vi "Actor Receive.vi"(11 "Process in":refnum<class "ABD.lvclass">) -> (0 "error out":errorcluster, 2 "Msg":refnum<class "Msg Strategy.lvclass">)   [LabVIEW 2021, in "ABD.lvlib" / "ABD.lvclass"]
uses:
  ABD.lvclass
  LVCAM/LVCAM/Msg Strategy/Msg Strategy.lvclass
  ABD.lvclass/ABD.ctl
  LVCAM/LVCAM/Actor/Actor.lvclass
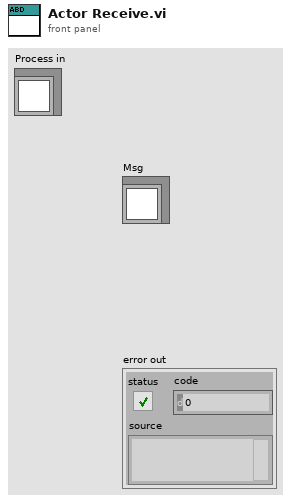
[diagram p1: front panel]
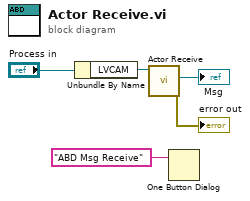
[diagram p0: block diagram]
diagram:
  n1 = Unbundle By Name("Process in") -> ("LVCAM"=w2:refnum<class "Actor.lvclass">)
  n2 = call-dynamic "Actor Receive.vi"("Actor in"=w2) -> ("error out"=→"error out":errorcluster, "Msg"=→"Msg":refnum<class "Msg Strategy.lvclass">)  [unwired: 9 in]
  n3 = One Button Dialog(message="ABD Msg Receive") -> ()  [unwired: 1 in, 1 out]
